vi "Set User Status.vi"(8 "error in (no error)":errorcluster, 10 "Value":bool, 11 "VISA resource name in":refnum<visa-resource-name>) -> (0 "error out":errorcluster, 3 "VISA resource name":refnum<visa-resource-name>)   [LabVIEW 2024, in "CTIPicoVISA.lvlib"]
doc: "Sets the onboard LED, if present, to the specified value. The status source will automatically be set to User which will disable any active status sources, such as communication (Comms)."
uses:
  CTIPicoVISA.lvlib
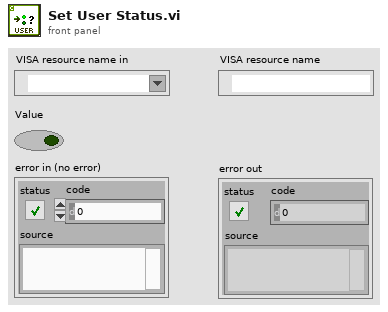
[diagram p1: front panel]
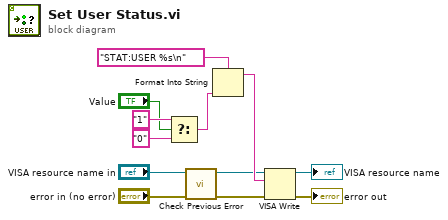
[diagram p0: block diagram]
diagram:
  n1 = Select(t="1", s="Value", f="0") -> (s? t:f=w11:string)
  n2 = call "Check Previous Error.vi"("error in (no error)"="error in (no error)", "VISA resource name in"="VISA resource name in") -> ("error out"=w8:errorcluster, "VISA resource name"=w9:refnum<visa-resource-name>)  [unwired: 8 in]
  n3 = Format Into String(format string="STAT:USER %s\n", w11) -> (resulting string=w10:string)  [unwired: 2 in, 1 out]
  n4 = VISA Write(VISA resource name=w9, write buffer=w10, error in (no error)=w8) -> (VISA resource name out=→"VISA resource name":refnum<visa-resource-name>, error out=→"error out":errorcluster)  [unwired: 1 out]
